vi "Read N Images from Buffer.vi"(8 "error in":errorcluster, 9 "timeout (-1 = wait forever)":i32 format="%d ms", 10 "count (-1 = all)":i32=-1, 11 "IRead Images in":refnum<class "IRead Image.lvclass">) -> (0 "error out":errorcluster, 2 "images":refnum<class "Generic Image.lvclass">[](array[class]), 3 "IRead Images out":refnum<class "IRead Image.lvclass">)   [LabVIEW 2024, in "IRead Image.lvclass"]
uses:
  IRead Image.lvclass
  Typedefs/Generic Image/Generic Image.lvclass
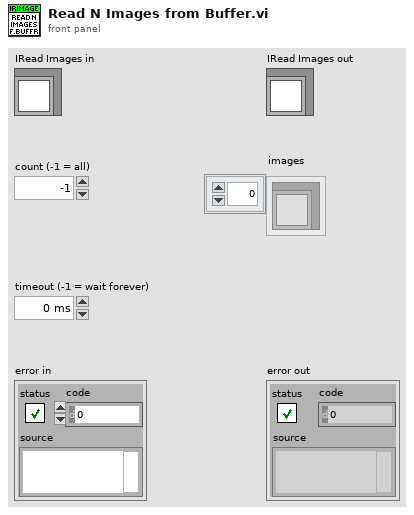
[diagram p1: front panel]
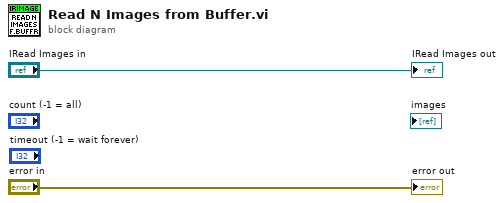
[diagram p0: block diagram]
diagram:
  "error out" <- "error in"
  "IRead Images out" <- "IRead Images in"
